vi "EJERCICIO 8.vi"() -> ()   [LabVIEW 2014]
panel:
  out "XY Graph":cluster{"Y":dbl[], "Y":dbl[]}[](graph)
  out "RMS SEÑAL 2":dbl(knob) scale=0.0..1000.0
  out "RMS SEÑAL 1":dbl(knob) scale=0.0..1000.0
  in  "?":bool
  out "Señal 2":dynamicdata(graph)
  in  "?":T1 {"Fase 2" scale=0.0..90.0; "Frecuencia 2" scale=0.0..500.0; "Amplitud 2" scale=0.0..1000.0}
  out "Señal 1":dynamicdata(graph)
  in  "?":T2 {"Fase 1" scale=0.0..90.0; "Frecuencia 1" scale=0.0..500.0; "Amplitud 1" scale=0.0..1000.0}
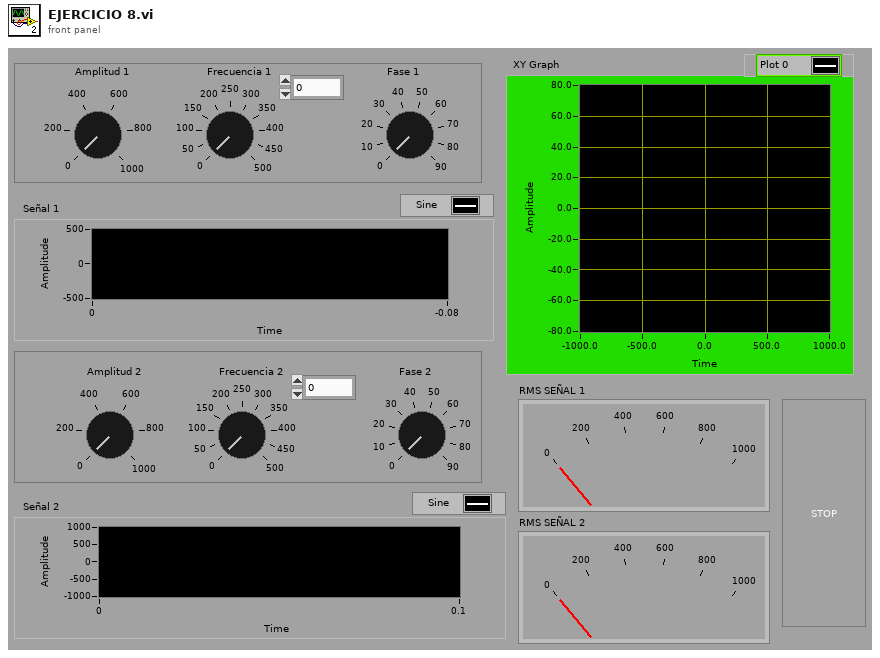
[diagram p1: front panel]
types:
  T1 = cluster{"Amplitud 2":dbl, "Frecuencia 2":dbl, "Fase 2":dbl}
  T2 = cluster{"Amplitud 1":dbl, "Frecuencia 1 ":dbl, "Fase 1 ":dbl}
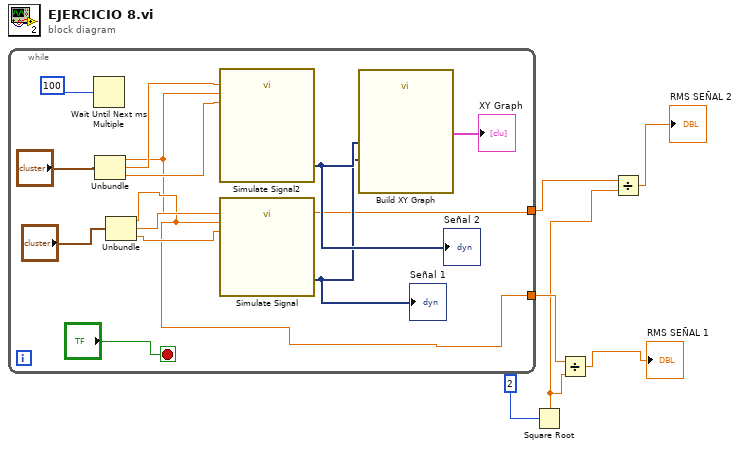
[diagram p0: block diagram]
diagram:
  n1 = while {
    tunnel: [w8] -> w6
    tunnel: [w7] -> w4
    stop <- "?" stop-if-true
    n2 = Wait Until Next ms Multiple(millisecond multiple=100) -> ()  [unwired: 1 out]
    n3 = Unbundle "Unbundle"("?") -> ("Amplitud 2"=w7:dbl, "Frecuencia 2"=w10:dbl, "Fase 2"=w11:dbl)
    n4 = Unbundle("?") -> ("Amplitud 1"=w8:dbl, "Frecuencia 1"=w18:dbl, "Fase 1"=w9:dbl)
    n5 = call "Simulate Signal2"("Frequency"=w10, "Amplitude"=w7, "Phase"=w11) -> ("Sine"=w14:dynamicdata)  [unwired: 11 in, 1 out]
    "Señal 2" <- w14
    n6 = call "Simulate Signal"("Frequency"=w18, "Amplitude"=w8, "Phase"=w9) -> ("Sine"=w13:dynamicdata)  [unwired: 11 in, 1 out]
    "Señal 1" <- w13
    n7 = call "Build XY Graph"("Y Input"=w13, "X Input"=w14) -> ("XY Graph"=→"XY Graph":cluster{"Y":dbl[], "Y":dbl[]}[])  [unwired: 3 in, 6 out]
  }
  n8 = Square Root(x=2) -> (sqrt(x)=w2:dbl)
  n9 = Divide(x=w6, y=w2) -> (x/y=→"RMS SEÑAL 1":dbl)
  n10 = Divide(x=w4, y=w2) -> (x/y=→"RMS SEÑAL 2":dbl)
